vi "SingleMotorPID.vi"(8 "PID constants":dbl[](array[numeric]), 9 "Max Rate":dbl, 10 "Actual":dbl, 11 "Target":dbl) -> (3 "Output":dbl)   [LabVIEW 2014]
panel:
  out "x+y":dbl
  out "s? t:f":dbl
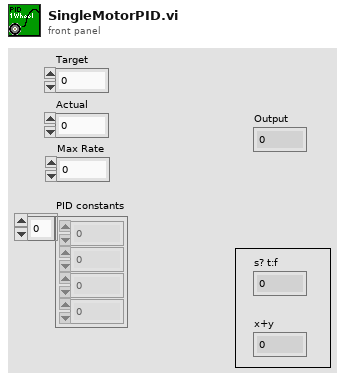
[diagram p1: front panel]
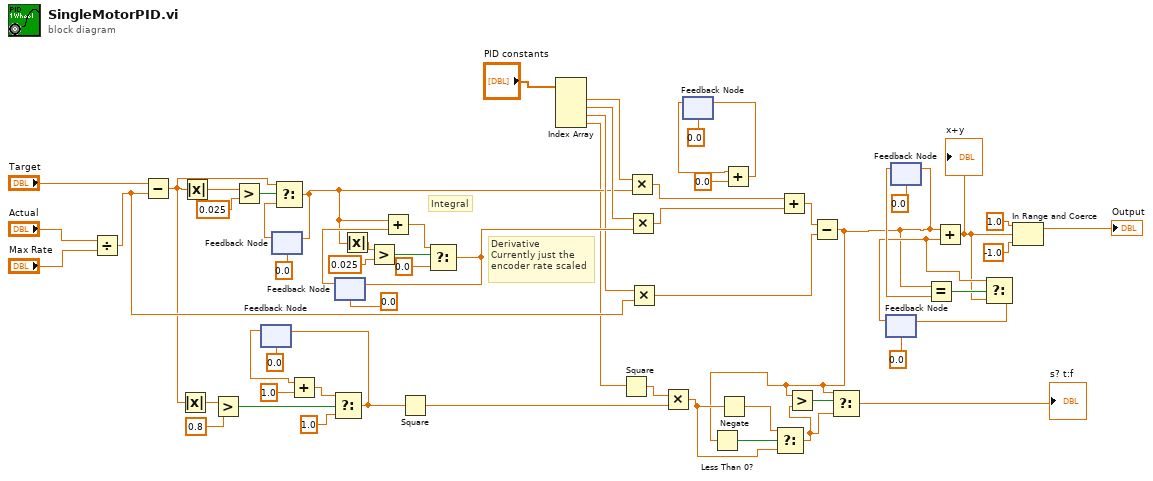
[diagram p0: block diagram]
diagram:
  # "Derivative\nCurrently just the\nencoder rate scaled"
  # "Integral"
  n1 = Divide(x="Actual", y="Max Rate") -> (x/y=w49:dbl)
  n2 = Subtract(x="Target", y=w49) -> (x-y=w27:dbl)
  n3 = Absolute Value(x=w27) -> (abs(x)=w29:dbl)
  n4 = Absolute Value(x=w27) -> (abs(x)=w39:dbl)
  n5 = Greater?(x=w29, y=0.8) -> (0:w26:bool)
  n6 = Greater?(x=w39, y=0.025) -> (0:w42:bool)
  n7 = feedback #1(0.0) -> (w24:dbl)
  n8 = feedback #2(0.0) -> (w41:dbl)
  n9 = Select(t=w27, s=w42, f=w41) -> (s? t:f=w37:dbl)
  n10 = feedback-in #2(w37) -> ()
  n11 = Add(x=w24, y=1.0) -> (x+y=w23:dbl)
  n12 = Select(t=w23, s=w26, f=1.0) -> (s? t:f=w21:dbl)
  n13 = feedback-in #1(w21) -> ()
  n14 = feedback #3(0.0) -> (w52:dbl)
  n15 = Absolute Value(x=w37) -> (abs(x)=w38:dbl)
  n16 = Greater?(x=w38, y=0.025) -> (0:w55:bool)
  n17 = Add(x=w37, y=w52) -> (x+y=w54:dbl)
  n18 = Square(x=w21) -> (x^2=w20:dbl)
  n19 = Select(t=w54, s=w55, f=0.0) -> (s? t:f=w53:dbl)
  n20 = feedback-in #3(w53) -> ()
  n21 = Index Array(array="PID constants") -> (element #1=w46:dbl, element #2=w45:dbl, element #3=w44:dbl, element #4=w13:dbl)  [unwired: 4 in]
  n22 = Square(x=w13) -> (x^2=w12:dbl)
  n23 = Multiply(x=w46, y=w37) -> (x*y=w11:dbl)
  n24 = Multiply(x=w45, y=w53) -> (x*y=w59:dbl)
  n25 = Multiply(x=w44, y=w49) -> (x*y=w60:dbl)
  n26 = Multiply(x=w12, y=w20) -> (x*y=w16:dbl)
  n27 = feedback #4(0.0) -> (w31:dbl)
  n28 = Negate(x=w16) -> (-x=w17:dbl)
  n29 = Add(x=w31, y=0.0) -> (x+y=w30:dbl)
  n30 = feedback-in #4(w30) -> ()
  n31 = Add(x=w11, y=w59) -> (x+y=w58:dbl)
  n32 = Subtract(x=w58, y=w60) -> (x-y=w1:dbl)
  n33 = Less Than 0?(x=w1) -> (x < 0?=w18:bool)
  n34 = Select(t=w17, s=w18, f=w16) -> (s? t:f=w15:dbl)
  n35 = Greater?(x=w1, y=w15) -> (0:w19:bool)
  n36 = Select(t=w1, s=w19, f=w15) -> (s? t:f=→"s? t:f":dbl)
  n37 = feedback #5(0.0) -> (w6:dbl)
  n38 = feedback-in #6(w1) -> ()
  n39 = feedback #6(0.0) -> (w8:dbl)
  n40 = Equal?(x=w1, y=w8) -> (x = y?=w7:bool)
  n41 = Add(x=w1, y=w6) -> (x+y=w4:dbl)
  "x+y" <- w4
  n42 = Select(t=w6, s=w7, f=w4) -> (s? t:f=w5:dbl)
  n43 = feedback-in #5(w5) -> ()
  n44 = In Range and Coerce(upper limit=1.0, x=w4, lower limit=-1.0) -> (coerced(x)=→"Output":dbl)  [unwired: 1 out]
